vi "get Names.vi"(8 "error in (no error)":errorcluster, 11 "VI Collection in":refnum<class "VI Collection.lvclass">) -> (0 "error out":errorcluster, 1 "VI Ref":refnum<vi>[](array[refnum]), 2 "VI Names":string[](array[string]), 3 "VI Collection out":refnum<class "VI Collection.lvclass">)   [LabVIEW 2015, in "QuickVIew.lvlib" / "VI Collection.lvclass"]
doc: "TLB Prime - Application Template 1.3.0.24\nNorm Kirchner, NI Systems Engineering - NI\nCopyright (c) 2014, NI"
uses:
  VI Collection.lvclass
  VI Collection.lvclass/VI Collection.ctl
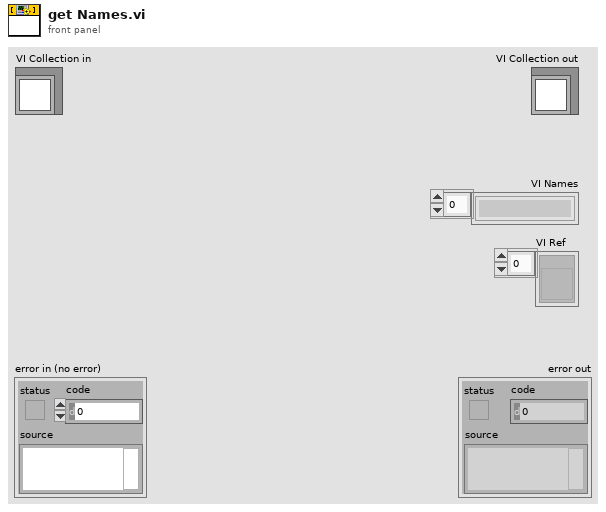
[diagram p1: front panel]
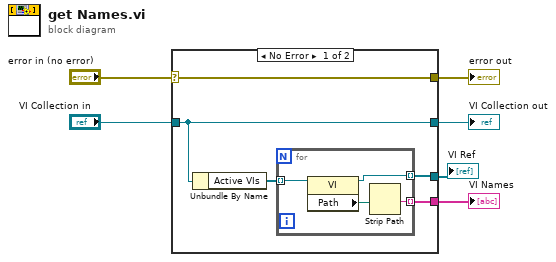
[diagram p0: block diagram]
diagram:
  n1 = case shown="No Error" "error in (no error)" {
    selector: "error in (no error)" -> [w10 w17]
    tunnel: [w10 w17] -> w5
    tunnel: [w11 w16] -> w3
    tunnel: "VI Collection in" -> [w11 w16]
    tunnel: [w8 _] -> w2
    tunnel: [w7 _] -> w1
    frame No Error {
      n2 = Unbundle By Name(w11) -> ("Active VIs"=w9:refnum<vi>[])
      n3 = for {
        tunnel: w9 -> [w15] mode=indexing
        tunnel: [w14] -> w8 mode=indexing
        tunnel: [w12] -> w7 mode=indexing
        n4 = property class="VI"(reference=w15) -> (reference out=w12:refnum<vi>, "Path"=w13:path)  [unwired: 1 in, 1 out]
        n5 = Strip Path(path=w13) -> (name=w14:string)  [unwired: 1 out]
      }
    }
    frame Error {
    }
  }
  "error out" <- w5
  "VI Collection out" <- w3
  "VI Names" <- w2
  "VI Ref" <- w1
